vi "SVFA Unit Conversion (Complex) (N Ch).vi"(0 "complex spectra":T9(array[cluster]) {"spectrum info"."x-axis units" items=["Time (s)"=0, "Frequency-CB (Hz)"=1, "Frequency-CPB (Hz)"=1248, "Frequency-Arbitrary (Hz)"=2357, "Quefrency (s)"=2, "Revolutions (rev)"=3, "Order"=4, "Speed (RPM)"=11, "Speed (rad/s)"=21, "Index"=65535]; "spectrum info"."weighting filter" items=["Linear", "A-weighting", "B-weighting", "C-weighting", "ITU-R 468-4", "Dolby", "CCITT", "C-message", "Wb", "Wc", "Wd", "We", "Wf", "Wh", "Wj", "Wk", "Wm", "AES17 20 kHz lowpass", "AES17 40 kHz lowpass", "AES17 20 kHz highpass", "AES17 40 kHz highpass"]; "spectrum info"."dB reference [EU]" format="%.2f"; "spectrum info"."engineering units" items=["custom..."=0, "V"=1, "A"=21, "C"=30, "pC"=31, "s"=32, "-"=29, "Pa"=2, "N"=20, "g"=3, "m/s^2"=4, "m/s"=5, "m"=6, "mm/s"=12, "mm"=13, "micron/s"=14, "micron"=15, "in/s^2"=7, "in/s"=8, "in"=9, "mil/s"=10, "mil"=11, "rad/s^2"=16, "rad/s"=17, "rad"=18, "deg/s^2"=26, "deg/s"=27, "deg"=28, "RPM"=22, "cycle/s^2"=23, "Hz"=24, "cycle"=25, "strain"=19]; "spectrum info"."spectral info"."window" items=["None "=0, "Hanning"=1, "Hamming"=2, "Blackman-Harris"=3, "Exact Blackman"=4, "Blackman"=5, "Flat Top"=6, "4 Term B-Harris "=7, "7 Term B-Harris"=8, "Low Sidelobe"=9, "Force - Exponential"=10, "Gaussian"=62]; "complex spectrum"."complex spectrum" format="%.2f"; "complex spectrum"."dx" format="%.2f"; "complex spectrum"."x0" format="%.2f"}, 1 "desired scaling":T8 {"dB reference (0: no change)" format="%.2f"}, 2 "spectral density desired":T1(ring), 3 "unwrap phase (F)":bool, 4 "convert to degree (T)":bool=TRUE, 5 "error in (no error)":errorcluster) -> (14 "converted spectra":cluster{"x0":dbl, "dx":dbl, "magnitude":dbl[]}[](array[cluster]) {"magnitude" format="%.2p"; "dx" format="%.2p"; "x0" format="%.2p"}, 15 "magnitude unit labels":string[](array[string]), 16 "phase spectra":cluster{"x0":dbl, "dx":dbl, "phase":dbl[]}[](array[cluster]) {"phase" format="%.2p"; "dx" format="%.2p"; "x0" format="%.2p"}, 17 "phase unit labels":string[](array[string]), 18 "spectrum info out":T2[](array[typedef]) {"x-axis units" items=["Time (s)"=0, "Frequency-CB (Hz)"=1, "Frequency-CPB (Hz)"=1248, "Frequency-Arbitrary (Hz)"=2357, "Quefrency (s)"=2, "Revolutions (rev)"=3, "Order"=4, "Speed (RPM)"=11, "Speed (rad/s)"=21, "Index"=65535]; "weighting filter" items=["Linear", "A-weighting", "B-weighting", "C-weighting", "ITU-R 468-4", "Dolby", "CCITT", "C-message", "Wb", "Wc", "Wd", "We", "Wf", "Wh", "Wj", "Wk", "Wm", "AES17 20 kHz lowpass", "AES17 40 kHz lowpass", "AES17 20 kHz highpass", "AES17 40 kHz highpass"]; "dB reference [EU]" format="%.2f"; "engineering units" items=["custom..."=0, "V"=1, "A"=21, "C"=30, "pC"=31, "s"=32, "-"=29, "Pa"=2, "N"=20, "g"=3, "m/s^2"=4, "m/s"=5, "m"=6, "mm/s"=12, "mm"=13, "micron/s"=14, "micron"=15, "in/s^2"=7, "in/s"=8, "in"=9, "mil/s"=10, "mil"=11, "rad/s^2"=16, "rad/s"=17, "rad"=18, "deg/s^2"=26, "deg/s"=27, "deg"=28, "RPM"=22, "cycle/s^2"=23, "Hz"=24, "cycle"=25, "strain"=19]; "spectral info"."window" items=["None "=0, "Hanning"=1, "Hamming"=2, "Blackman-Harris"=3, "Exact Blackman"=4, "Blackman"=5, "Flat Top"=6, "4 Term B-Harris "=7, "7 Term B-Harris"=8, "Low Sidelobe"=9, "Force - Exponential"=10, "Gaussian"=62]}, 19 "error out":errorcluster)   [LabVIEW 2017]
doc: "Converts between dB/linear, magnitude/magnitude^2, rms/peak/peak-peak, spectrum/spectral density, and dB ref1/dB ref2. Wire data to the <B>spectrum</B> input to determine the polymorphic instance to use or manually select the instance."
uses:
  <vilib>/addons/_NISVFA/_Shared subVIs/Controls/svc_Spectrum Info.ctl
  <vilib>/addons/_NISVFA/_Shared subVIs/Controls/svc_X-Axis Units.ctl
  <vilib>/addons/_NISVFA/_Shared subVIs/Controls/svc_Spectrum Type.ctl
  <vilib>/addons/_NISVFA/_Shared subVIs/Controls/svc_Engineering Units Text Ring.ctl
  <vilib>/addons/_NISVFA/_Shared subVIs/Controls/svc_Weighting Filter Text Ring.ctl
  <vilib>/addons/_NISVFA/_Shared subVIs/Controls/svc_Complimentary Spectrum Units.ctl
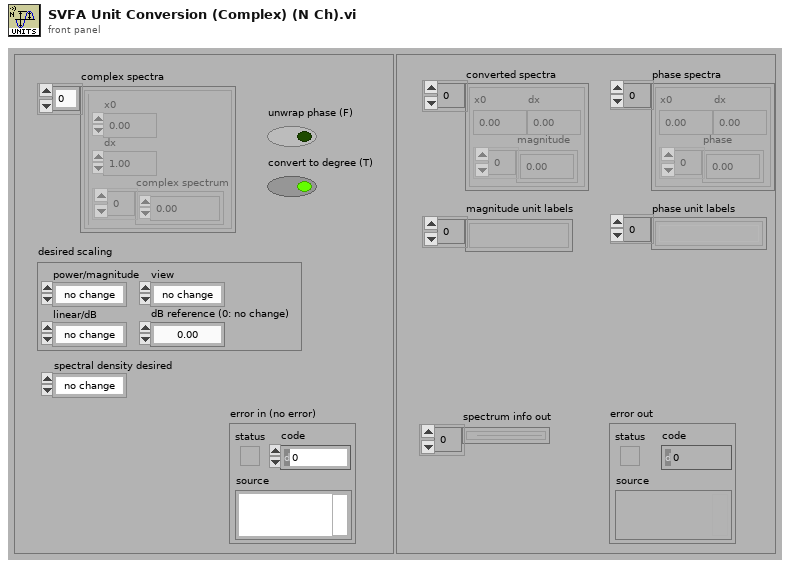
[diagram p1: front panel]
types:
  T1 = enum16{"no change", "spectrum", "spectral density"}
  T2 = typedef "svc_Spectrum Info.ctl" = cluster{"channel name":string, "description":string, "x-axis units":T3, "spectral info":cluster{"spectrum type":T4, "linear/dB":enum16{"linear", "dB"}, "window":u16, "window size":i32, "FFT size":i32}, "engineering units":T5, "custom label":string, "dB reference [EU]":dbl, "peak units":enum16{"rms", "peak", "peak-peak"}, "weighting filter":T6, "spectral density?":bool, "unit label":string, "spectrum skewed?":bool, "complimentary spectrum units":T7}
  T3 = typedef "svc_X-Axis Units.ctl" = u16
  T4 = typedef "svc_Spectrum Type.ctl" = enum16{"FFT Spectrum [complex]", "Amplitude [Magnitude]", "Power [Magnitude^2]", "Cross Spectrum [complex]", "Frequency Response [Complex]"}
  T5 = typedef "svc_Engineering Units Text Ring.ctl" = u16
  T6 = typedef "svc_Weighting Filter Text Ring.ctl" = u16
  T7 = typedef "svc_Complimentary Spectrum Units.ctl" = enum16{"none", "radians", "degrees", "cycles", "imaginary"}
  T8 = cluster{"linear/dB":enum16{"no change", "linear", "dB"}, "dB reference (0: no change)":dbl, "power/magnitude":enum16{"no change", "power", "magnitude"}, "view":enum16{"no change", "rms", "peak", "peak-peak"}}
  T9 = cluster{"complex spectrum":cluster{"x0":dbl, "dx":dbl, "complex spectrum":cdb[]}, "spectrum info":T2}[]
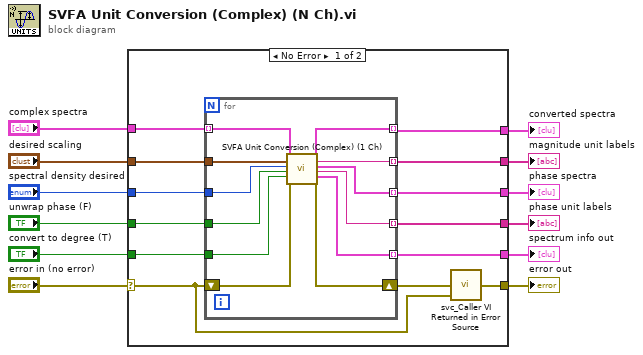
[diagram p0: block diagram]
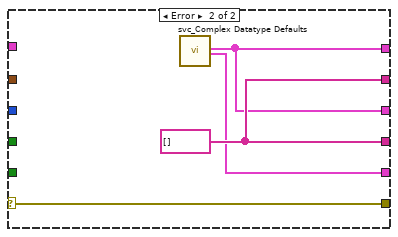
[diagram p2: hidden frame]
diagram:
  n1 = case shown="No Error" "error in (no error)" {
    selector: "error in (no error)" -> [w13 w41]
    tunnel: "complex spectra" -> [w25 _]
    tunnel: "desired scaling" -> [w24 _]
    tunnel: [w19 w41] -> w10
    tunnel: [w22 w39] -> w9
    tunnel: [w21 w38] -> w8
    tunnel: [w20 w40] -> w7
    tunnel: [w18 w39] -> w5
    tunnel: [w17 w40] -> w4
    tunnel: "convert to degree (T)" -> [w16 _]
    tunnel: "unwrap phase (F)" -> [w15 _]
    tunnel: "spectral density desired" -> [w14 _]
    frame No Error {
      n2 = for {
        tunnel: [w37] -> w22 mode=indexing
        shift-right: [w36] -> w23
        shift-left: w13 -> [w35]
        tunnel: w25 -> [w34] mode=indexing
        tunnel: w24 -> [w33]
        tunnel: [w32] -> w21 mode=indexing
        tunnel: [w31] -> w20 mode=indexing
        tunnel: [w30] -> w18 mode=indexing
        tunnel: [w29] -> w17 mode=indexing
        tunnel: w16 -> [w28]
        tunnel: w15 -> [w27]
        tunnel: w14 -> [w26]
        n3 = call <vilib>:"SVFA Unit Conversion (Complex) (1 Ch).vi"("complex spectrum"=w34, "desired scaling"=w33, "spectral density desired"=w26, "unwrap phase (F)"=w27, "convert to degree (T)"=w28, "error in (no error)"=w35) -> ("converted spectrum"=w37:cluster{"x0":dbl, "dx":dbl, "magnitude":dbl[]}, "magnitude unit label"=w31:string, "phase spectrum"=w30:cluster{"x0":dbl, "dx":dbl, "phase":dbl[]}, "phase unit label"=w29:string, "spectrum info out"=w32:T2, "error out"=w36:errorcluster)  [unwired: 8 in]
      }
      n4 = call <vilib>:"svc_Caller VI Returned in Error Source.vi"("warning input to caller"=w13, "error in (no error)"=w23) -> ("error out"=w19:errorcluster)  [unwired: 3 in]
    }
    frame Error {
      w40 = string[] []
      n5 = call <vilib>:"svc_Complex Datatype Defaults.vi"() -> ("empty array of spectra"=w39:cluster{"f0":dbl, "df":dbl, "magnitude":dbl[]}[], "empty array of spectrum info"=w38:T2[])  [unwired: 11 in, 7 out]
    }
  }
  "error out" <- w10
  "spectrum info out" <- w8
  "converted spectra" <- w9
  "magnitude unit labels" <- w7
  "phase spectra" <- w5
  "phase unit labels" <- w4
